vi "Get JSON Array Bounds.vi"(9 "invalid in":bool, 10 "Index":i32=-1, 11 "tokens":cluster{"token type":T1, T2}[](array[cluster])) -> (3 "array of JSON objects":T4[](array[typedef]))   [LabVIEW 2020, in "Multi Error Cluster.lvlib"]
doc: "Given tokens desribing a JSON array, describe the top level elements."
uses:
  <vilib>/MultiError/TokenizeJSON/Multi Error Cluster.lvlib
  <vilib>/MultiError/Errors Cluster Multiple Errors/JSON Object Descriptor.ctl
  <vilib>/MultiError/Errors Cluster Multiple Errors/JSON Token Descriptor.ctl
  <vilib>/MultiError/TokenizeJSON/JSON Raw Token Values.ctl
  <vilib>/MultiError/TokenizeJSON/JSON Token Values.ctl
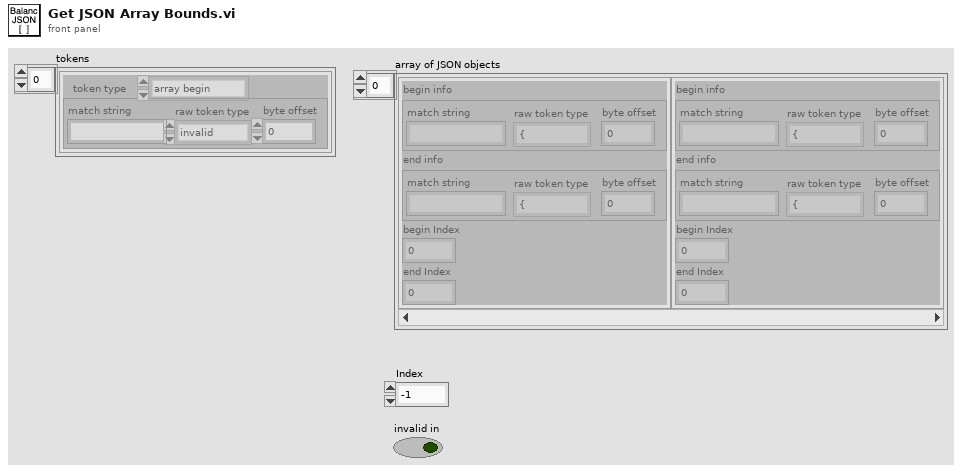
[diagram p1: front panel]
types:
  T1 = typedef "Multi Error Cluster.lvlib/JSON Token Values.ctl" = enum32{"array begin", "array end", "object begin", "object end", "value", "invalid", "name"}
  T2 = typedef "Multi Error Cluster.lvlib/JSON Token Descriptor.ctl" = cluster{"match string":string, "raw token type":T3, "byte offset ":i32}
  T3 = typedef "Multi Error Cluster.lvlib/JSON Raw Token Values.ctl" = enum32{"{", "}", "[", "]", ",", ":", "\"", "number", "string", "true", "false", "null", "invalid"}
  T4 = typedef "Multi Error Cluster.lvlib/JSON Object Descriptor.ctl" = cluster{"begin info":T2, "end info":T2, "begin Index":i32, "end Index":i32}
  T5 = cluster{cluster{"whole match":string, "raw token type":T3, "offset past match":i32}, cluster{"whole match":string, "raw token type":T3, "offset past match":i32}, "begin Index":i32, "end Index":i32}
  T6 = cluster{cluster{"whole match":string, "raw token type":T3, "offset past match":i32}, cluster{"whole match":string, "raw token type":T3, "offset past match":i32}, "begin Index":i32, "end Index":i32}[]
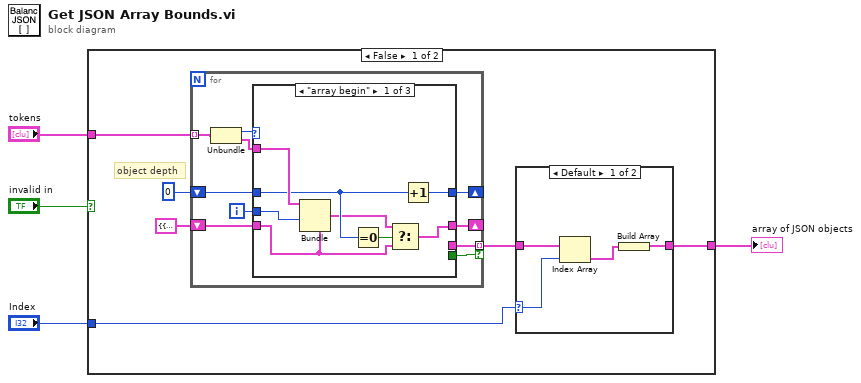
[diagram p0: block diagram]
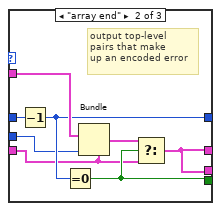
[diagram p3: hidden frame]
diagram:
  n1 = case shown="False" "invalid in" {
    tunnel: "tokens" -> [w8 _]
    tunnel: "Index" -> [w7 _]
    tunnel: [w5 _] -> w2
    frame False {
      # "object depth"
      n2 = for {
        tunnel: w8 -> [w25] mode=indexing
        shift-right: [w22] -> _
        shift-left: 0 -> [w23]
        shift-right: [w19] -> _
        shift-left: T5 {{"whole match"="", "raw token type"=enum."{", "offset past match"=0}, {"whole match"="", "raw token type"=enum."}", "offset past match"=0}, "begin Index"=-1, "end Index"=-1} -> [w21]
        tunnel: [w18] -> w6 mode=indexing if=w17
        i -> [w16]
        n3 = Unbundle(w25) -> ("token type"=w24:T1, w20:T2)
        n4 = case shown="\"array begin\"" w24 {
          tunnel: w23 -> [w31 w41 w43]
          tunnel: [w33 w39 w43] -> w22
          tunnel: w21 -> [w29 w36 w42]
          tunnel: w20 -> [w32 w40 _]
          tunnel: [w27 w35 w42] -> w19
          tunnel: [_ w35 _] -> w18
          tunnel: [_ w38 _] -> w17
          tunnel: w16 -> [w26 w34 _]
          frame "array begin" {
            n5 = Bundle(cluster=w29, w32, "begin Index"=w26) -> (w28:T5)  [unwired: 2 in]
            n6 = Equal To 0?(x=w31) -> (x = 0?=w30:bool)
            n7 = Select(t=w28, s=w30, f=w29) -> (s? t:f=w27:T5)
            n8 = Increment(x=w31) -> (x+1=w33:i32)
          }
          frame "array end" {
            # "output top-level\npairs that make\nup an encoded error"
            n9 = Decrement(x=w41) -> (x-1=w39:i32)
            n10 = Equal To 0?(x=w39) -> (x = 0?=w38:bool)
            n11 = Bundle(cluster=w36, w40, "end Index"=w34) -> (w37:T5)  [unwired: 2 in]
            n12 = Select(t=w37, s=w38, f=w36) -> (s? t:f=w35:T5)
          }
          frame Default {
          }
        }
      }
      n13 = case shown="Default" w7 {
        selector: w7 -> [w13 _]
        tunnel: w6 -> [w14 w15]
        tunnel: [w11 w15] -> w5
        frame Default {
          n14 = Index Array(array=w14, index=w13) -> (element=w12:T5)
          n15 = Build Array(w12) -> (w11:T6)
        }
        frame -1 {
        }
      }
    }
    frame True {
    }
  }
  "array of JSON objects" <- w2
